vi "Pumpensteuerung_PID.vi"(4 "reinitialize? (F)":bool, 7 "PID Regelung Pumpe":bool, 9 "FI13 SW in l/min":dbl, 10 "Prozessvariable":dbl, 11 "Pumpensteuerung":dbl) -> (1 "Regeldifferenz":dbl, 2 "?":dbl, 3 "upper limit":dbl)   [LabVIEW 2015]
uses:
  <vilib>/addons/control/pid/pid.llb/PID (DBL).vi
  <vilib>/addons/control/pid/NI_PID_pid.lvlib
panel:
  in  "PID gains":T1={"proportional gain (Kc)"=0.12, "integral time (Ti, min)"=0.16, "derivative time (Td, min)"=0.0} {"derivative time (Td, min)" format="%.3f"; "integral time (Ti, min)" format="%.3f"; "proportional gain (Kc)" format="%.3f"}
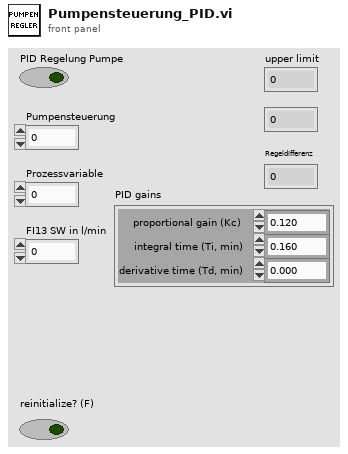
[diagram p1: front panel]
types:
  T1 = cluster{"proportional gain (Kc)":dbl, "integral time (Ti, min)":dbl, "derivative time (Td, min)":dbl}
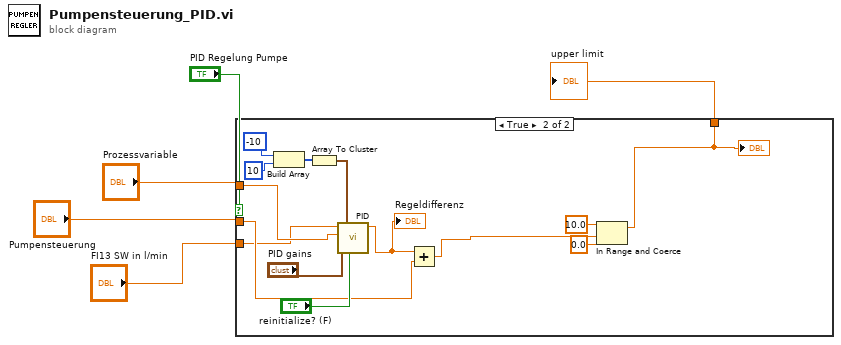
[diagram p0: block diagram]
diagram:
  n1 = case shown="True" "PID Regelung Pumpe" {
    tunnel: "Pumpensteuerung" -> [w6 w17]
    tunnel: "Prozessvariable" -> [_ w19]
    tunnel: "FI13 SW in l/min" -> [_ w12]
    tunnel: [w6 w11] -> w5
    frame False {
    }
    frame True {
      n2 = Build Array(-10, 10) -> (w15:i32[])
      n3 = Array To Cluster(array=w15) -> (cluster=w16:cluster{"[0]":i32, "[1]":i32})
      n4 = call-poly <vilib>:"PID.vi"("reinitialize? (F)"="reinitialize? (F)", "output range"=w16, "PID gains"="PID gains", "process variable"=w19, "setpoint"=w12) -> ("output"=w18:dbl)  [unwired: 5 in, 1 out]
      "Regeldifferenz" <- w18
      n5 = Add(x=w18, y=w17) -> (x+y=w10:dbl)
      n6 = In Range and Coerce(upper limit=10.0, x=w10, lower limit=0.0) -> (coerced(x)=w11:dbl)  [unwired: 1 out]
      "?" <- w11
    }
  }
  "upper limit" <- w5
